vi "GetV.vi"(0 "VISA resource name":refnum<visa-resource-name>) -> (2 "VISA resource name out":refnum<visa-resource-name>, 3 "output 1":dbl)   [LabVIEW 2020]
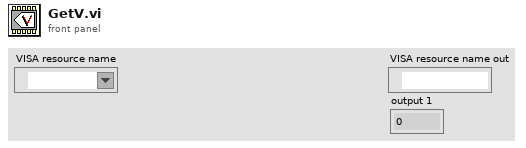
[diagram p1: front panel]
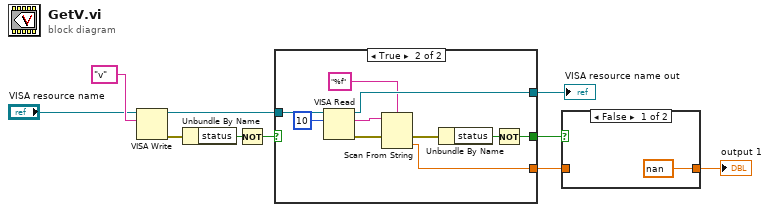
[diagram p0: block diagram]
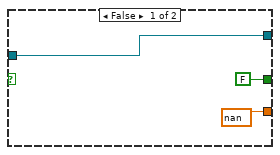
[diagram p2: hidden frame]
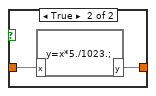
[diagram p3: hidden frame]
diagram:
  n1 = VISA Write(VISA resource name="VISA resource name", write buffer="v") -> (VISA resource name out=w3:refnum<visa-resource-name>, error out=w1:errorcluster)  [unwired: 1 in, 1 out]
  n2 = Unbundle By Name(w1) -> ("status"=w2:bool)
  n3 = Not(x=w2) -> (.not. x?=w5:bool)
  n4 = case shown="True" w5 {
    tunnel: [w11 w23] -> w8
    tunnel: [nan w18] -> w7
    tunnel: [FALSE w17] -> w6
    tunnel: w3 -> [w11 w16]
    frame False {
    }
    frame True {
      n5 = VISA Read(VISA resource name=w16, byte count=u32 10) -> (VISA resource name out=w23:refnum<visa-resource-name>, read buffer=w20:string, error out=w19:errorcluster)  [unwired: 1 in, 1 out]
      n6 = Scan From String(format string="%f", input string=w20, error in=w19) -> (error out=w15:errorcluster, output 1=w18:dbl)  [unwired: 2 in, 2 out]
      n7 = Unbundle By Name(w15) -> ("status"=w14:bool)
      n8 = Not(x=w14) -> (.not. x?=w17:bool)
    }
  }
  "VISA resource name out" <- w8
  n9 = case shown="False" w6 {
    tunnel: w7 -> [_ w26]
    tunnel: [nan w25] -> w9
    frame False {
    }
    frame True {
      n10 = formula code="y=x*5./1023.;"("x"=w26) -> ("y"=w25:dbl)
    }
  }
  "output 1" <- w9
